vi "XY Graph Get Tail or Head Fraction.vi"(8 "Tail (F)/Head (T)":bool, 9 "Array Index":dbl, 10 "Peak Index":dbl, 11 "X Array":dbl[](array[numeric])) -> (1 "Head or Tail Fraction":dbl)   [LabVIEW 2021, in "XY Graph Add-Ons.lvlib"]
doc: "Given an array with a maximum (peak) and a fractional index, returns what fraction of the head or tail the index corresponds to."
uses:
  XY Graph Add-Ons.lvlib
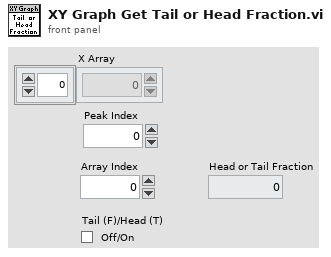
[diagram p1: front panel]
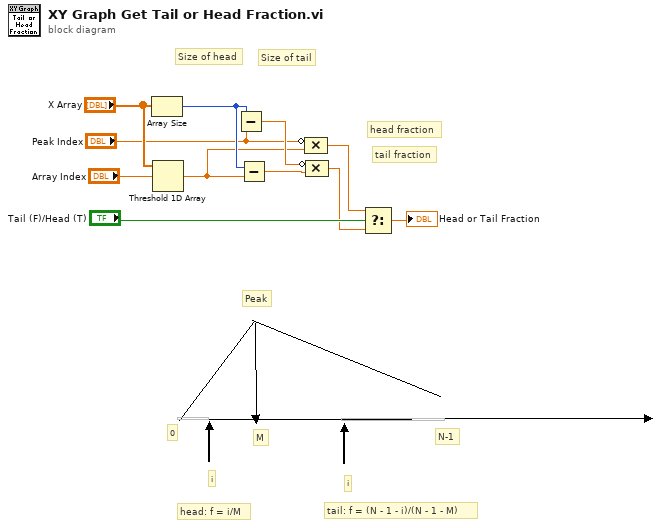
[diagram p0: block diagram]
diagram:
  # "tail: f = (N - 1 - i)/(N - 1 - M)"
  # "i"
  # "head: f = i/M"
  # "i"
  # "M"
  # "N-1"
  # "0"
  # "Peak"
  # "tail fraction"
  # "head fraction"
  # "Size of head"
  # "Size of tail"
  n1 = Array Size(array="X Array") -> (size(s)=w3:i32)
  n2 = Threshold 1D Array(2:"Array Index", 3:"X Array") -> (0:w2:dbl)  [unwired: 1 in]
  n3 = Subtract(x=w3, y="Peak Index") -> (x-y=w6:dbl)
  n4 = Subtract(x=w3, y=w2) -> (x-y=w7:dbl)
  n5 = Compound Arithmetic op=MULTIPLY(invert "Peak Index", w2) -> (w8:dbl)
  n6 = Compound Arithmetic op=MULTIPLY(invert w6, w7) -> (w5:dbl)
  n7 = Select(t=w8, s="Tail (F)/Head (T)", f=w5) -> (s? t:f=→"Head or Tail Fraction":dbl)
